vi "Send_User_Event_Polymorphic.vi"   [LabVIEW 2014, in "User_Event_Library.lvlib"]
uses:
  User_Event_Library.lvlib
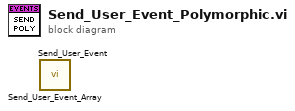
[diagram p0: block diagram]
diagram:
  n1 = call "Send_User_Event_Array.vi"() -> ()  [unwired: 10 in, 2 out]
  n2 = call "Send_User_Event.vi"() -> ()  [unwired: 10 in, 2 out]
